vi "Delete Recipe.vi"(8 "error in (no error)":errorcluster, 10 "index":i32, 11 "Master in":refnum<class "Master.lvclass">) -> (0 "error out":errorcluster, 3 "Master out":refnum<class "Master.lvclass">)   [LabVIEW 2014, in "Master.lvclass"]
uses:
  Master/Master.lvclass
  Master/Master.lvclass/Master.ctl
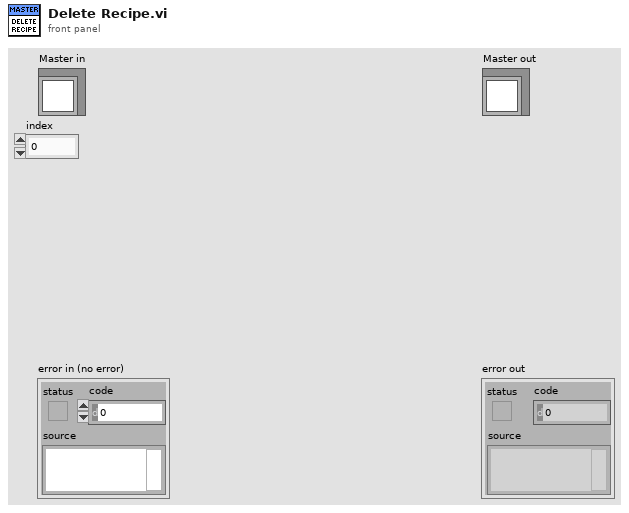
[diagram p1: front panel]
types:
  T1 = cluster{"Name":string, "Wind Length":string, "Wind Spd":string, "Kink Cyc":string, "Bind Length":string, "Unit":string}[]
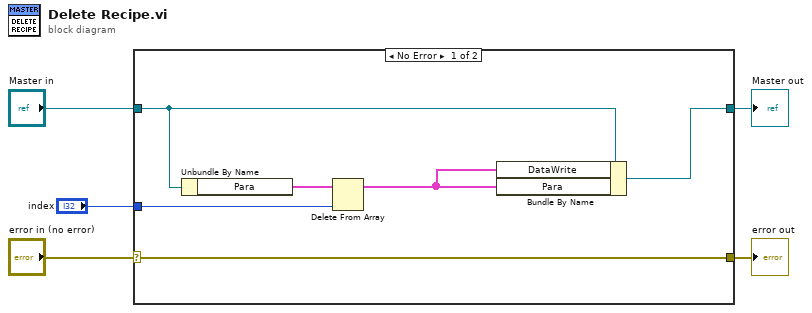
[diagram p0: block diagram]
diagram:
  n1 = case shown="No Error" "error in (no error)" {
    selector: "error in (no error)" -> [w11 w13]
    tunnel: [w11 w13] -> w4
    tunnel: [w6 w12] -> w2
    tunnel: "Master in" -> [w8 w12]
    tunnel: "index" -> [w9 _]
    frame No Error {
      n2 = Unbundle By Name(w8) -> ("Para"=w10:T1)
      n3 = Delete From Array(array=w10, index=w9) -> (array with subset deleted=w7:T1)  [unwired: 1 in, 1 out]
      n4 = Bundle By Name(cluster=w8, "DataWrite"=w7, "Para"=w7) -> (w6:refnum<class "Master.lvclass">)
    }
    frame Error {
    }
  }
  "error out" <- w4
  "Master out" <- w2
